vi "Untitled 4.vi"() -> ()   [LabVIEW 2020]
panel:
  out "output 2":i32
  in  "String 2":string
  out "output 1":string
  in  "String":string
  out "length":i32
  out "data":string
  out "value":variant
  out "data string":string
  out "variant out":variant
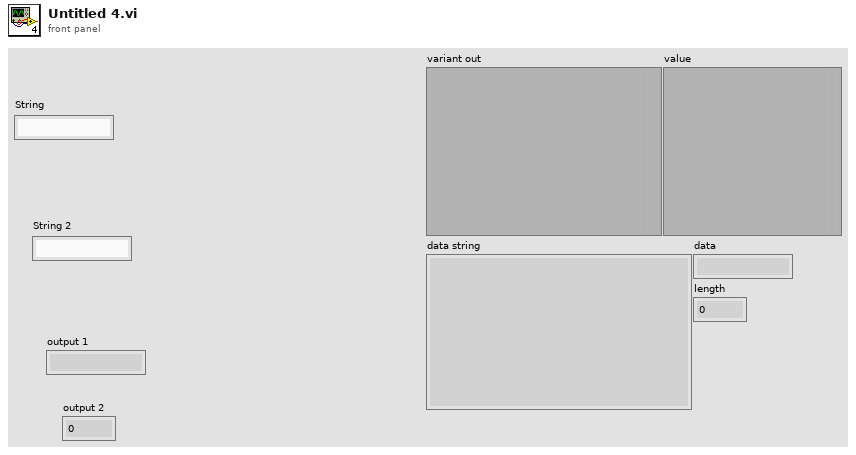
[diagram p1: front panel]
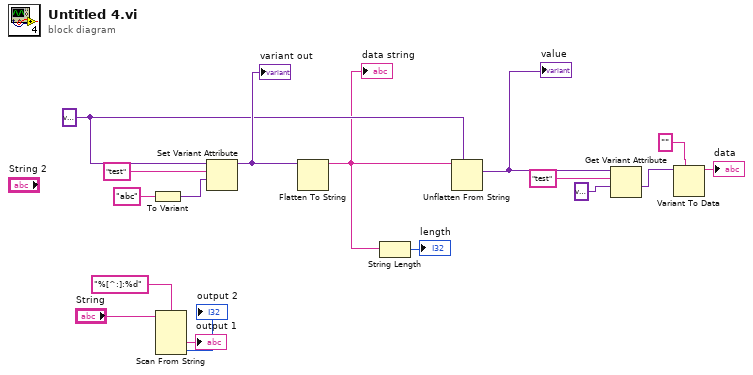
[diagram p0: block diagram]
diagram:
  w13 = variant
  n1 = To Variant(anything="abc") -> (Variant=w15:variant)
  n2 = Scan From String(format string="%[^:]:%d", input string="String") -> (output 1=→"output 1":string, output 2=→"output 2":i32)  [unwired: 4 in, 3 out]
  n3 = Set Variant Attribute(Variant=w13, name="test", value=w15) -> (Variant out=w14:variant)  [unwired: 1 in, 2 out]
  "variant out" <- w14
  n4 = Flatten To String(anything=w14) -> (data string=w6:string)  [unwired: 3 in, 2 out]
  "data string" <- w6
  n5 = String Length(string=w6) -> (length=→"length":i32)
  n6 = Unflatten From String(type=w13, binary string=w6) -> (value=w12:variant)  [unwired: 3 in, 2 out]
  "value" <- w12
  n7 = Get Variant Attribute(Variant=w12, name="test", default value (empty Variant)=variant) -> (value=w9:variant)  [unwired: 1 in, 3 out]
  n8 = Variant To Data(type="", Variant=w9) -> (data=→"data":string)  [unwired: 1 in, 1 out]
